vi "_PC_D999 data_collapse.vi"(8 "error in (no error)":errorcluster, 10 "data cluster in":T2, 11 "Refnum cluster in":T1) -> (0 "error out":errorcluster, 3 "Refnum cluster out":T1)   [LabVIEW 2018]
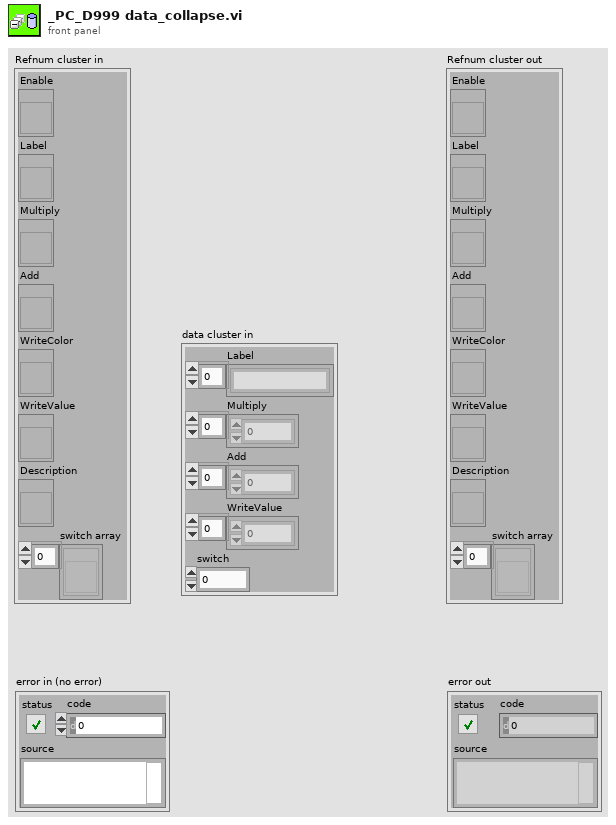
[diagram p1: front panel]
types:
  T1 = cluster{"Enable":refnum<vi>, "Label":refnum<vi>, "Multiply":refnum<vi>, "Add":refnum<vi>, "WriteColor":refnum<vi>, "WriteValue":refnum<vi>, "Description":refnum<vi>, "switch array":refnum<vi>[]}
  T2 = cluster{"Label":string[], "Multiply":dbl[], "Add":dbl[], "WriteValue":i16[], "switch":u32}
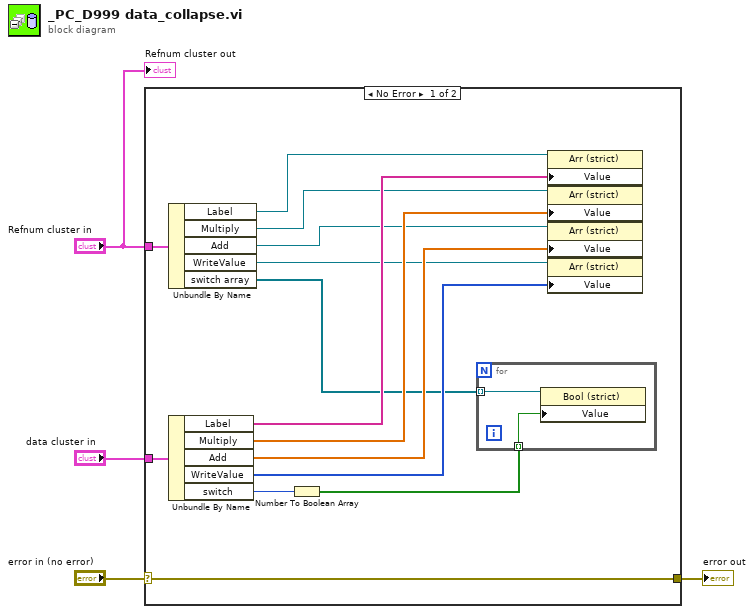
[diagram p0: block diagram]
diagram:
  n1 = case shown="No Error" "error in (no error)" {
    selector: "error in (no error)" -> [w8 w21]
    tunnel: "Refnum cluster in" -> [w18 _]
    tunnel: "data cluster in" -> [w17 _]
    tunnel: [w8 w21] -> w2
    frame No Error {
      n2 = Unbundle By Name(w18) -> ("Label"=w12:refnum<vi>, "Multiply"=w11:refnum<vi>, "Add"=w10:refnum<vi>, "WriteValue"=w9:refnum<vi>, "switch array"=w6:refnum<vi>[])
      n3 = Unbundle By Name(w17) -> ("Label"=w16:string[], "Multiply"=w15:dbl[], "Add"=w14:dbl[], "WriteValue"=w13:i16[], "switch"=w7:u32)
      n4 = Number To Boolean Array(number=w7) -> (Boolean array=w5:bool[])
      n5 = for {
        tunnel: w6 -> [w20] mode=indexing
        tunnel: w5 -> [w19] mode=indexing
        n6 = property class="Bool (strict)"(reference=w20, "Value"=w19) -> ()  [unwired: 1 in, 2 out]
      }
      n7 = property class="Arr (strict)"(reference=w12, "Value"=w16) -> ()  [unwired: 1 in, 2 out]
      n8 = property class="Arr (strict)"(reference=w11, "Value"=w15) -> ()  [unwired: 1 in, 2 out]
      n9 = property class="Arr (strict)"(reference=w10, "Value"=w14) -> ()  [unwired: 1 in, 2 out]
      n10 = property class="Arr (strict)"(reference=w9, "Value"=w13) -> ()  [unwired: 1 in, 2 out]
    }
    frame Error {
    }
  }
  "error out" <- w2
  "Refnum cluster out" <- "Refnum cluster in"
